vi "D.vi"(1 "Promien krzywizny południka [v]":dbl, 2 "t":dbl, 3 "fi[rad]":dbl) -> (0 "D":dbl)   [LabVIEW 2015, in "Biblioteka moduł map v3.lvlib" / "Konwersja wsp.lvlib" / "UTM.lvlib" / "Konwersja na UTM.lvlib"]
doc: "Współczynnik wzoru na konwersję na UTM."
uses:
  Konwersja na UTM.lvlib
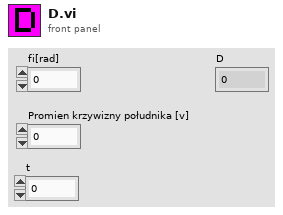
[diagram p1: front panel]
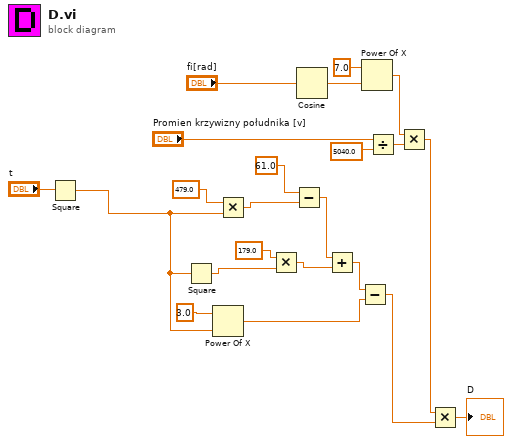
[diagram p0: block diagram]
diagram:
  n1 = Square(x="t") -> (x^2=w4:dbl)
  n2 = Square(x=w4) -> (x^2=w5:dbl)
  n3 = Power Of X(1:w4, 2:3.0 ("y")) -> (0:w2:dbl)
  n4 = Multiply(x=479.0 ("y"), y=w4) -> (x*y=w10:dbl)
  n5 = Multiply(x=179.0 ("y"), y=w5) -> (x*y=w7:dbl)
  n6 = Subtract(x=61.0 ("y"), y=w10) -> (x-y=w9:dbl)
  n7 = Cosine(x="fi[rad]") -> (cos(x)=w17:dbl)
  n8 = Add(x=w9, y=w7) -> (x+y=w6:dbl)
  n9 = Subtract(x=w6, y=w2) -> (x-y=w1:dbl)
  n10 = Power Of X(1:w17, 2:7.0 ("y")) -> (0:w19:dbl)
  n11 = Divide(x="Promien krzywizny południka [v]", y=5040.0) -> (x/y=w20:dbl)
  n12 = Multiply(x=w19, y=w20) -> (x*y=w21:dbl)
  n13 = Multiply(x=w21, y=w1) -> (x*y=→"D":dbl)
